vi "initialise.vi"(8 "error in (no error)":errorcluster, 11 "GenericPlugin in":refnum<class "FPGAWrapperMM140723Galvo.lvclass">) -> (0 "error out":errorcluster, 3 "GenericPlugin out":refnum<class "FPGAWrapperMM140723Galvo.lvclass">)   [LabVIEW 2010, in "FPGAWrapperMM140723Galvo.lvclass"]
doc: "The dynamic dispatch-version of this VI initalises the plug-in object by allocating and initalising any dynamic resources need."
uses:
  FPGAWrapperMM140723Galvo.lvclass
  GenericFPGAWrapper/GenericFPGAWrapper/GenericFPGAWrapper.lvclass
  type definitions/command_enum.ctl
  FPGAWrapperMM140723Galvo.lvclass/FPGAWrapperMM140723Galvo.ctl
  class_data.vi
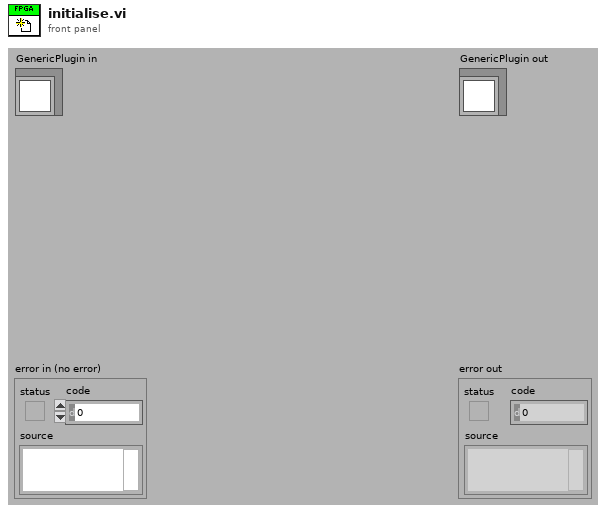
[diagram p1: front panel]
types:
  T1 = typedef "command_enum.ctl" = enum16{"NULL", "update", "start", "stop", "reset", "shut-down"}
  T2 = typedef "config_data_cluster.ctl" = cluster{"bit file":string, "hifo box version":i32, "ADC clock phase":i32}
  T3 = typedef "settings_cluster.ctl" = cluster{"number of pixels":i64, "pixel frequency (Hz)":dbl, "pixel values cluster":T4, "triggered?":bool, "triggered flag valid?":bool, "gates":T5[]}
  T4 = typedef "channels_cluster.ctl" = cluster{"channel 0":u32, "channel 1":u32, "channel 2":u32, "channel 3":u32}
  T5 = typedef "gate_cluster.ctl" = cluster{"index":i32, "parameters":T6}
  T6 = typedef "gate_parameters_cluster.ctl" = cluster{"offset":i64, "pulsing":i64, "not pulsing":i64, "cycles per pulse":i64, "repetitions":i64}
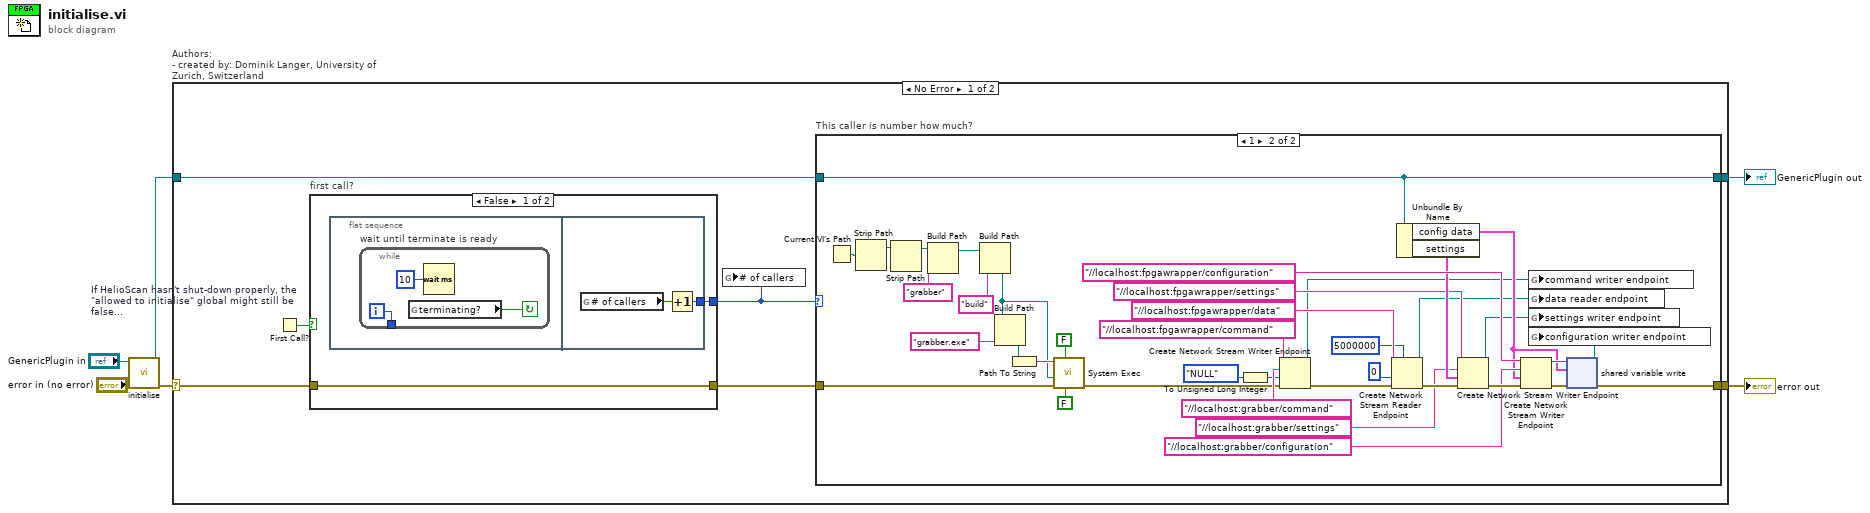
[diagram p0: block diagram]
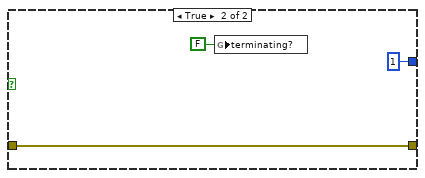
[diagram p2: hidden frame]
diagram:
  n1 = call-parent "initialise.vi"("error in (no error)"="error in (no error)", "GenericPlugin in"="GenericPlugin in") -> ("error out"=w4:errorcluster, "GenericPlugin out"=w3:refnum<class "FPGAWrapperMM140723Galvo.lvclass">)  [unwired: 8 in]
  n2 = case "Authors: \n- created by: Dominik Langer, University of Zurich, Switzerland" shown="No Error" w4 {
    selector: w4 -> [w10 w64]
    tunnel: w3 -> [w9 w65]
    tunnel: [w13 w64] -> w2
    tunnel: [w12 w65] -> w1
    frame No Error {
      n3 = First Call? "If HelioScan hasn't shut-down properly, the \"allowed to initialise\" global might still be false..."() -> (First Call?: T/F=w11:bool)
      n4 = case "first call?" shown="False" w11 {
        tunnel: [w15 1 ("# of callers")] -> w7
        tunnel: [w14 w22] -> w8
        tunnel: w10 -> [w14 w22]
        frame False {
          n5 = flat-sequence {
            tunnel: [w19] -> w15
            frame #0 {
              n6 = while "wait until terminate is ready" {
                tunnel: [w16] -> _
                i -> [w16]
                stop <- w18 continue-if-true
                n7 = global read "class_data.vi" "terminating?"() -> (w18:bool)
                n8 = Wait (ms)(milliseconds to wait=u32 10) -> ()  [unwired: 1 out]
              }
            }
            frame #1 {
              n9 = global read "class_data.vi" "# of callers"() -> (w20:i32)
              n10 = Increment(x=w20) -> (x+1=w19:i32)
            }
          }
        }
        frame True {
          n11 = global write "class_data.vi" "terminating?"(FALSE ("ready for initialise?")) -> ()
        }
      }
      n12 = global write "class_data.vi" "# of callers"(w7) -> ()
      n13 = case "This caller is number how much?" shown="1" w7 {
        tunnel: w8 -> [w24 w62]
        tunnel: [w25 w61] -> w12
        tunnel: w9 -> [w25 w61]
        tunnel: [w24 w63] -> w13
        frame Default {
          # "It's not the first caller, so we don't have to initialise (has already been done)..."
        }
        frame 1 {
          n14 = Current VI's Path() -> (path=w41:path)
          n15 = Strip Path(path=w41) -> (stripped path=w42:path)  [unwired: 1 out]
          n16 = Strip Path(path=w42) -> (stripped path=w43:path)  [unwired: 1 out]
          n17 = Build Path(base path=w43, name or relative path="grabber") -> (appended path=w29:path)
          n18 = Build Path(base path=w29, name or relative path="build") -> (appended path=w28:path)
          n19 = Build Path(base path=w28, name or relative path="grabber.exe" ("command line")) -> (appended path=w38:path)
          n20 = Path To String(path=w38) -> (string=w39:string)
          n21 = call <vilib>:"System Exec.vi"("run minimized? (F)"=FALSE, "wait until completion? (T)"=FALSE, "error in (no error)"=w62, "working directory"=w28, "command line"=w39) -> ("error out"=w40:errorcluster)  [unwired: 3 in, 3 out]
          n22 = To Unsigned Long Integer(number=command_enum."NULL" ("command")) -> (unsigned 32bit integer=w58:u32)
          n23 = Create Network Stream Writer Endpoint(8:w40, 9:w58, 10:"//localhost:grabber/command" ("writer name"), 11:"//localhost:fpgawrapper/command" ("writer name")) -> (0:w56:errorcluster, 3:w35:refnum<k21>)  [unwired: 2 in]
          n24 = Create Network Stream Reader Endpoint(7:5000000 ("reader buffer size"), 8:w56, 9:u64 0, 11:"//localhost:fpgawrapper/data" ("reader url")) -> (0:w51:errorcluster, 3:w34:refnum<k21>)  [unwired: 2 in]
          n25 = Unbundle By Name(w61) -> ("config data"=w45:T2, "settings"=w52:T3)
          n26 = Create Network Stream Writer Endpoint(8:w51, 9:w52, 10:"//localhost:grabber/settings" ("writer name"), 11:"//localhost:fpgawrapper/settings" ("writer name")) -> (0:w50:errorcluster, 3:w33:refnum<k21>)  [unwired: 2 in]
          n27 = Create Network Stream Writer Endpoint(8:w50, 9:w45, 10:"//localhost:grabber/configuration" ("reader url"), 11:"//localhost:fpgawrapper/configuration" ("writer name")) -> (0:w53:errorcluster, 3:w54:refnum<k21>)  [unwired: 2 in]
          n28 = global write "class_data.vi" "command writer endpoint"(w35) -> ()
          n29 = global write "class_data.vi" "data reader endpoint"(w34) -> ()
          n30 = global write "class_data.vi" "settings writer endpoint"(w33) -> ()
          n31 = shared-variable-write(w54, w53, w45) -> (w26:refnum<k21>, w63:errorcluster)  [unwired: 1 in, 1 out]
          n32 = global write "class_data.vi" "configuration writer endpoint"(w26) -> ()
        }
      }
    }
    frame Error {
    }
  }
  "error out" <- w2
  "GenericPlugin out" <- w1
